vi "application time stamp.vi"(3 "VI Path":path) -> (0 "last mod":timestamp, 1 "this version":path)   [LabVIEW 2011, in "Design Server.lvlib"]
uses:
  Design Server.lvlib
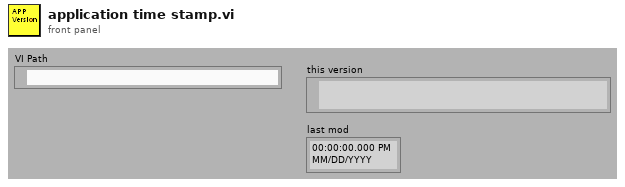
[diagram p1: front panel]
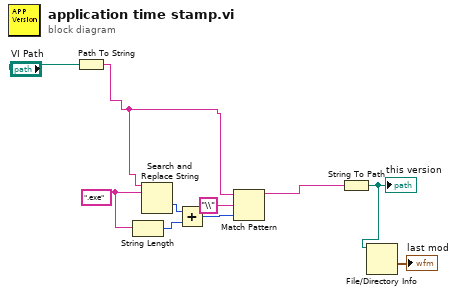
[diagram p0: block diagram]
diagram:
  w10 = ".exe" ("search string")
  n1 = Path To String(path="VI Path") -> (string=w2:string)
  n2 = String Length(string=w10) -> (length=w8:i32)
  n3 = Search and Replace String(input string=w2, search string=w10) -> (offset past replacement=w9:i32)  [unwired: 6 in, 3 out]
  n4 = Add(x=w9, y=w8) -> (x+y=w7:i32)
  n5 = Match Pattern(string=w2, regular expression="\\" ("search string"), offset (0)=w7) -> (before substring=w5:string)  [unwired: 3 out]
  n6 = String To Path(string=w5) -> (path=w4:path)
  "this version" <- w4
  n7 = File/Directory Info(path=w4) -> (last mod=→"last mod":timestamp)  [unwired: 1 in, 6 out]
